vi "Format Client Request (Notification).vi"(8 "error in (no error)":errorcluster, 9 "id":string, 10 "JSON Value in":variant, 11 "method":string) -> (0 "error out":errorcluster, 2 "Request String":string)   [LabVIEW 2020, in "JSON-RPC Lib.lvlib" / "JSONRPC Client.lvclass"]
uses:
  JSONRPC Client.lvclass
  Variant JSON API/Variant JSON API.lvlib
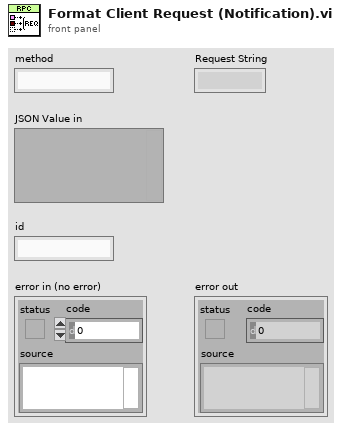
[diagram p1: front panel]
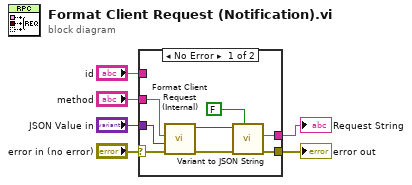
[diagram p0: block diagram]
diagram:
  n1 = case shown="No Error" "error in (no error)" {
    selector: "error in (no error)" -> [w14 w15]
    tunnel: [w13 w15] -> w5
    tunnel: "JSON Value in" -> [w8 _]
    tunnel: [w12 _] -> w3
    tunnel: "method" -> [w11 _]
    tunnel: "id" -> [_ _]
    frame No Error {
      n2 = call "Format Client Request (Internal).vi"("error in (no error)"=w14, "params"=w8, "method"=w11) -> ("error out"=w10:errorcluster, "JSON Value out"=w9:variant)  [unwired: 7 in]
      n3 = call "Variant to JSON String.vi"("pretty print? (F)"=FALSE ("pretty print? (T)"), "error in (no error)"=w10, "Variant in"=w9) -> ("error out"=w13:errorcluster, "String"=w12:string)  [unwired: 6 in, 1 out]
    }
    frame Error {
    }
  }
  "error out" <- w5
  "Request String" <- w3
